vi "Bert_or_Ernie.vi"() -> ()   [LabVIEW 2014]
panel:
  in  "On Bert?":bool
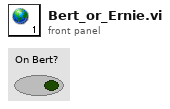
[diagram p1: front panel]
diagram:
